vi "test CompareFace.vi"() -> ()   [LabVIEW 2020]
uses:
  FaceRecognitionDotNet/FaceRecognition Class/FaceRecognition.lvclass
panel:
  out "CompareFace":bool
  out "Numeric":i32
  in  "stop":bool
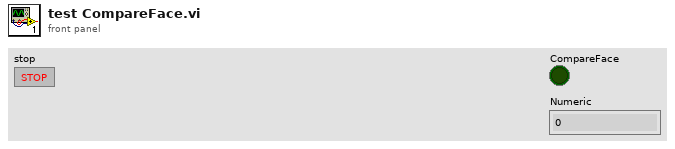
[diagram p1: front panel]
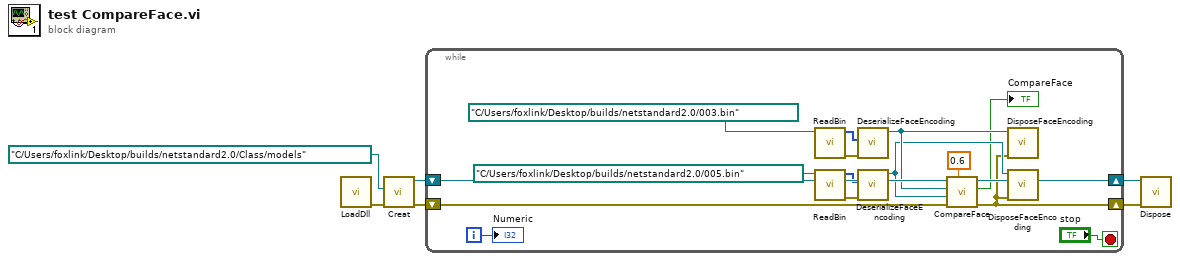
[diagram p0: block diagram]
diagram:
  n1 = call "LoadDll.vi"() -> ("error out"=w6:errorcluster)  [unwired: 11 in]
  n2 = call "Creat.vi"("error in (no error)"=w6, "mode path"=path "C:/Users/foxlink/Desktop/builds/netstandard2.0/Class/models") -> ("error out"=w2:errorcluster, "FaceRecognition out"=w5:refnum<class "FaceRecognition.lvclass">)  [unwired: 8 in]
  n3 = while {
    shift-right: [w21] -> w4
    shift-left: w5 -> [w22]
    shift-right: [w9] -> w3
    shift-left: w2 -> [w20]
    i -> [w18]
    stop <- "stop" stop-if-true
    n4 = call "ReadBin.vi"("FaceEncoding file"=path "C:/Users/foxlink/Desktop/builds/netstandard2.0/003.bin" ("path")) -> ("error out"=w16:errorcluster, "Array"=w15:u8[])  [unwired: 9 in]
    n5 = call "ReadBin.vi"("FaceEncoding file"=path "C:/Users/foxlink/Desktop/builds/netstandard2.0/005.bin" ("path")) -> ("error out"=w17:errorcluster, "Array"=w14:u8[])  [unwired: 9 in]
    n6 = call "DeserializeFaceEncoding.vi"("error in (no error)"=w16, "BinaryEncoding"=w15) -> ("FaceEncoding"=w11:refnum<k24>)  [unwired: 8 in, 1 out]
    n7 = call "DeserializeFaceEncoding.vi"("error in (no error)"=w17, "BinaryEncoding"=w14) -> ("FaceEncoding"=w10:refnum<k24>)  [unwired: 8 in, 1 out]
    n8 = call "CompareFace.vi"("tolerance"=0.6, "error in (no error)"=w20, "faceEncodingToCheck"=w10, "knownFaceEncoding"=w11, "FaceRecognition in"=w22) -> ("error out"=w9:errorcluster, "CompareFace"=→"CompareFace":bool, "FaceRecognition out"=w21:refnum<class "FaceRecognition.lvclass">)  [unwired: 4 in]
    n9 = call "DisposeFaceEncoding.vi"("error in (no error)"=w9, "FaceEncoding in"=w11) -> ()  [unwired: 9 in, 1 out]
    n10 = call "DisposeFaceEncoding.vi"("error in (no error)"=w9, "FaceEncoding in"=w10) -> ()  [unwired: 9 in, 1 out]
    "Numeric" <- w18
  }
  n11 = call "Dispose.vi"("error in (no error)"=w3, "FaceRecognition in"=w4) -> ()  [unwired: 8 in, 2 out]
